vi "CreateCursor.vi"(8 "Error In":errorcluster caption="错误输入", 10 "类型":enum16{"单光标", "双光标", "峰值光标", "无光标"}(ring), 11 "WaveformGraph输入":refnum<vi>) -> (0 "Error In 2":errorcluster caption="错误输入")   [LabVIEW 2012, in "WaveGraphX.xctl"]
uses:
  WaveGraphX.xctl
  <vilib>/Utility/miscctls.llb/LVCursorListTypeDef.ctl
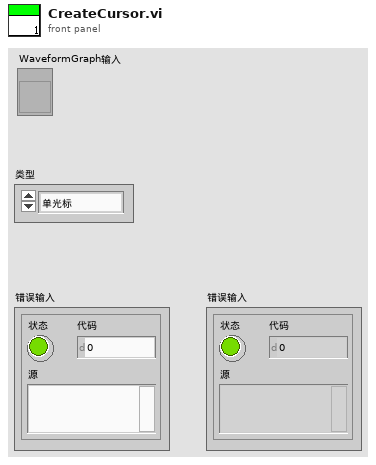
[diagram p1: front panel]
types:
  T1 = typedef "LVCursorListTypeDef.ctl" = cluster{"Name":string, "Color":u32, "Style":u8, "Point Style":u8, "Name Visible":bool, "Allow Drag":bool, "Cursor Mode":u32, "Plot":i32, "Index":i32, "Position":cluster{"X":dbl, "Y":dbl}, "X Scale":u32, "Y Scale":u32, "Watch Plots":i32[], "Watch All Plots":bool, "Plot Area":i32, "Label Offset":cluster{"X":dbl, "Y":dbl}}[]
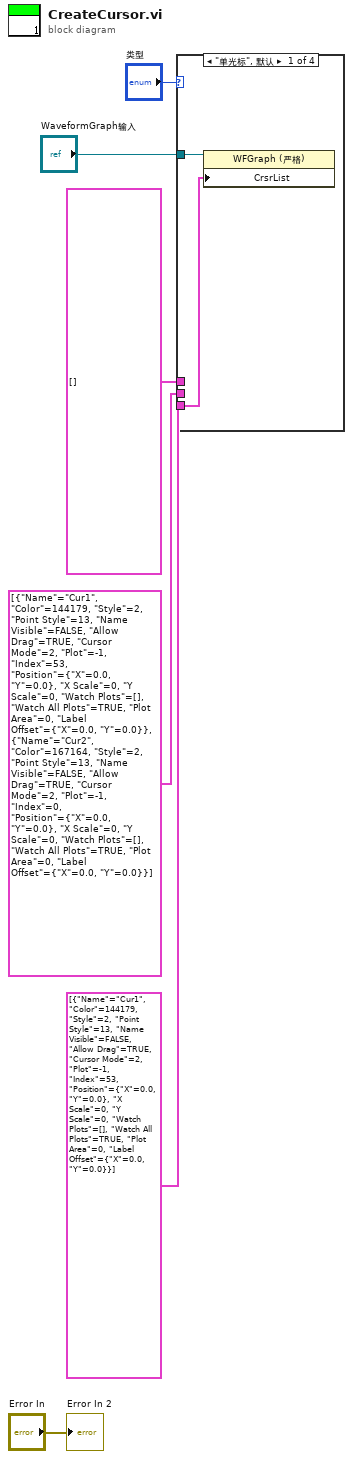
[diagram p0: block diagram]
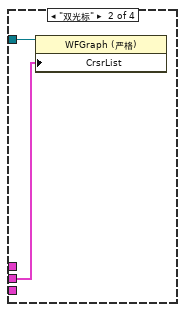
[diagram p2: hidden frame]
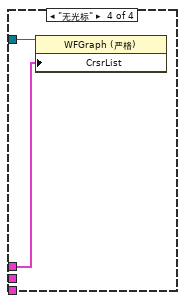
[diagram p4: hidden frame]
diagram:
  n1 = case shown="\"单光标\", 默认" "类型" {
    tunnel: "WaveformGraph输入" -> [w7 w10 _ w11]
    tunnel: T1 [{"Name"="Cur1", "Color"=144179, "Style"=2, "Point Style"=13, "Name Visible"=FALSE, "Allow Drag"=TRUE, "Cursor Mode"=2, "Plot"=-1, "Index"=53, "Position"={"X"=0.0, "Y"=0.0}, "X Scale"=0, "Y Scale"=0, "Watch Plots"=[], "Watch All Plots"=TRUE, "Plot Area"=0, "Label Offset"={"X"=0.0, "Y"=0.0}}, {"Name"="Cur2", "Color"=167164, "Style"=2, "Point Style"=13, "Name Visible"=FALSE, "Allow Drag"=TRUE, "Cursor Mode"=2, "Plot"=-1, "Index"=0, "Position"={"X"=0.0, "Y"=0.0}, "X Scale"=0, "Y Scale"=0, "Watch Plots"=[], "Watch All Plots"=TRUE, "Plot Area"=0, "Label Offset"={"X"=0.0, "Y"=0.0}}] ("游标列表") -> [_ w9 _ _]
    tunnel: T1 [{"Name"="Cur1", "Color"=144179, "Style"=2, "Point Style"=13, "Name Visible"=FALSE, "Allow Drag"=TRUE, "Cursor Mode"=2, "Plot"=-1, "Index"=53, "Position"={"X"=0.0, "Y"=0.0}, "X Scale"=0, "Y Scale"=0, "Watch Plots"=[], "Watch All Plots"=TRUE, "Plot Area"=0, "Label Offset"={"X"=0.0, "Y"=0.0}}] ("游标列表") -> [w8 _ _ _]
    tunnel: T1 [] ("游标列表") -> [_ _ _ w12]
    frame "单光标", Default {
      n2 = property class="WFGraph (严格)"(reference=w7, "CrsrList"=w8) -> ()  [unwired: 1 in, 2 out]
    }
    frame "双光标" {
      n3 = property class="WFGraph (严格)"(reference=w10, "CrsrList"=w9) -> ()  [unwired: 1 in, 2 out]
    }
    frame "峰值光标" {
    }
    frame "无光标" {
      n4 = property class="WFGraph (严格)"(reference=w11, "CrsrList"=w12) -> ()  [unwired: 1 in, 2 out]
    }
  }
  "Error In 2" <- "Error In"
